vi "ESC UART.vi"() -> (0 "error out":errorcluster)   [LabVIEW 2022 SP3]
doc: "This example performs writes and reads on a serial port, as directed by the user. You can press the Write and Read buttons, and change the Read Count, while the example is running.\n\nThe parameters set for the serial port must match the parameters of the connected instrument or device. In this example, the Read Count parameter specifies the number of bytes that the serial port reads. If there were more bytes at the port than the specified number, those bytes would not be read. If there were less bytes at the port than the specified number, you would receive a timeout error.\n\nThis example expands upon the flow control options for XON and XOFF, allowing the user to choose those control characters. Also, the user can enable or disable a termination character. Some devices require a termination character in order to identify the end of command strings. Some devices send a termination character to signify the end of data to be read. This example shows how you can end the Read operation once a termination character is detected in the buffer and/or append a termination character at the end of the Write data."
uses:
  Program Files/National Instruments/LabVIEW 2022/examples/Instrument IO/Serial/support/Serial - Settings.ctl
  Sub_vis/Upload Data.ctl
  Globals/Meas_global.vi
  <vilib>/Instr/_visa.llb/VISA Configure Serial Port (Instr).vi
panel:
  out "Port Number":string
  out "Sampling Freq Hz":dbl
  out "Status Flag":dbl
  out "Offset":i32
  out "unsigned byte array":u8[](array[numeric])
  out "No Of Errors":i32
  out "N Count":i32
  out "Happy":bool
  out "Status":bool
  out "Motor Duty Cycle":dbl
  out "Throttle Duty Cycle":dbl
  out "RPM":dbl
  out "Bus Current":dbl
  out "Voltage":dbl
  out "ESC Temperature":dbl
  in  "Read Count/ No. of Bytes":u32=22
  in  "Serial Settings":T1={"baud rate"=115200, "data bits"=8, "parity"=enum."None", "stop bits"=10, "flow control"=0} {"flow control" items=["None"=0, "XON/XOFF"=1, "RTS/CTS"=2, "DTR/DSR"=4]; "stop bits" items=["1.0"=10, "1.5"=15, "2.0"=20]; "data bits" min=5 max=8 step=1; "baud rate" items=["75"=75, "110"=110, "134"=134, "150"=150, "300"=300, "600"=600, "1200"=1200, "1800"=1800, "2400"=2400, "4800"=4800, "7200"=7200, "9600"=9600, "14400"=14400, "19200"=19200, "28800"=28800, "38400"=38400, "56000"=56000, "57600"=57600, "115200"=115200, "128000"=128000, "230400"=230400]}
  # "Overview: Reads ESC Data from UART Pins + FTDI Cable (Converts UART to Serial). \nAPD HV PRO 240a:\nNumber of Bytes = 22\nBaudrate 115200\nData Bits = 8\nParity = None\nStop Bits = 1.0\nFlow Control = None"
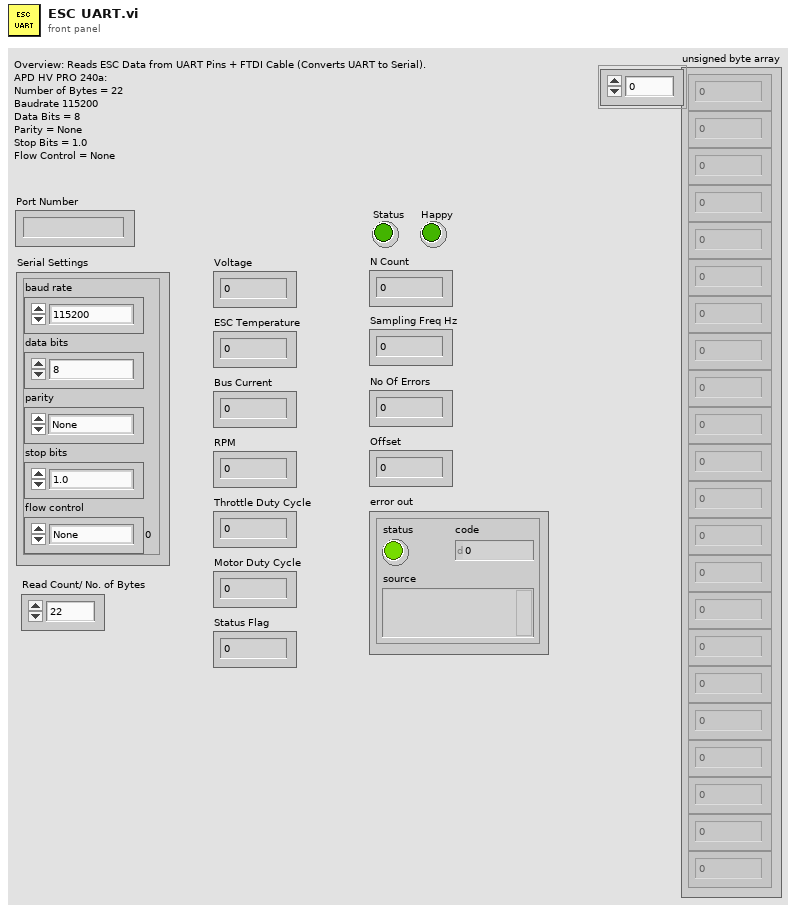
[diagram p1: front panel]
types:
  T1 = typedef "Serial - Settings.ctl" = cluster{"baud rate":u32, "data bits":u16, "parity":enum16{"None", "Odd", "Even", "Mark", "Space"}, "stop bits":u16, "flow control":u16}
  T2 = typedef "Setup.ctl" = enum16{"Run Program", "Show Setup", "Save Current Setup", "Setup Front Panel"}
  T3 = typedef "Upload Data.ctl" = enum16{"Voltage Array", "Time Trace Cluster"}
  T4 = typedef "Analysis_info_cluster.ctl" = cluster{"Colour":u32, "Inst type":T5, "Inst name":string, "Symbol":string, "Code name":string, "Extra Info":string, "Inst Array":T6, "Extra Titles":string[], "Extra Values":string[], "U":dbl, "u^2":dbl, "u^3":dbl, "u^4":dbl, "Skew_u":dbl, "Kurt_u":dbl, "Sd Error in Mean":dbl, "% u'/U":dbl, "X":dbl, "Y":dbl, "Z":dbl, "Timescale integral Estimate":dbl, "Sd Error in Variance":dbl, "Calib File":path, "Calib Constants":dbl[], "Output Position":bool, "Stats":enum16{"None", "Basic", "Full"}, "Av Sampling Rate":dbl, "Av No of Samples":dbl, "Total Meas Time (s)":dbl, "ADAM Ch Name":string, "Max value":dbl, "Min value":dbl, "Req Sample Rate Hz":dbl, "Sync Delay Time (s)":dbl, "Ch No":i16, "Device":string, "Use Latest Calib":bool, "Port":string, "Metadata Ch Names":string[], "Metadata Ch Values":string[], "Label":string}
  T5 = typedef "Inst_type.ctl" = enum16{"Raw voltage", "Raw with zero offsetting", "Propeller anemometer", "Pressure Transducer", "Pitot-static tube", "Hot wire", "Cross wire 1", "Cross wire 2", "Generic Linear", "Generic Polynomial", "Generic BackPoly", "Fast FID", "Thermocouple", "Cold wire", "Pulsed Wire", "LDA Vel", "LDA Tran time", "LDA Arr time", "Microphone"}
  T6 = typedef "Instrument_Array.ctl" = enum16{"PWA", "LDA", "Analogue"}
  T7 = typedef "Rendezvous RefNum" = refnum<k1>
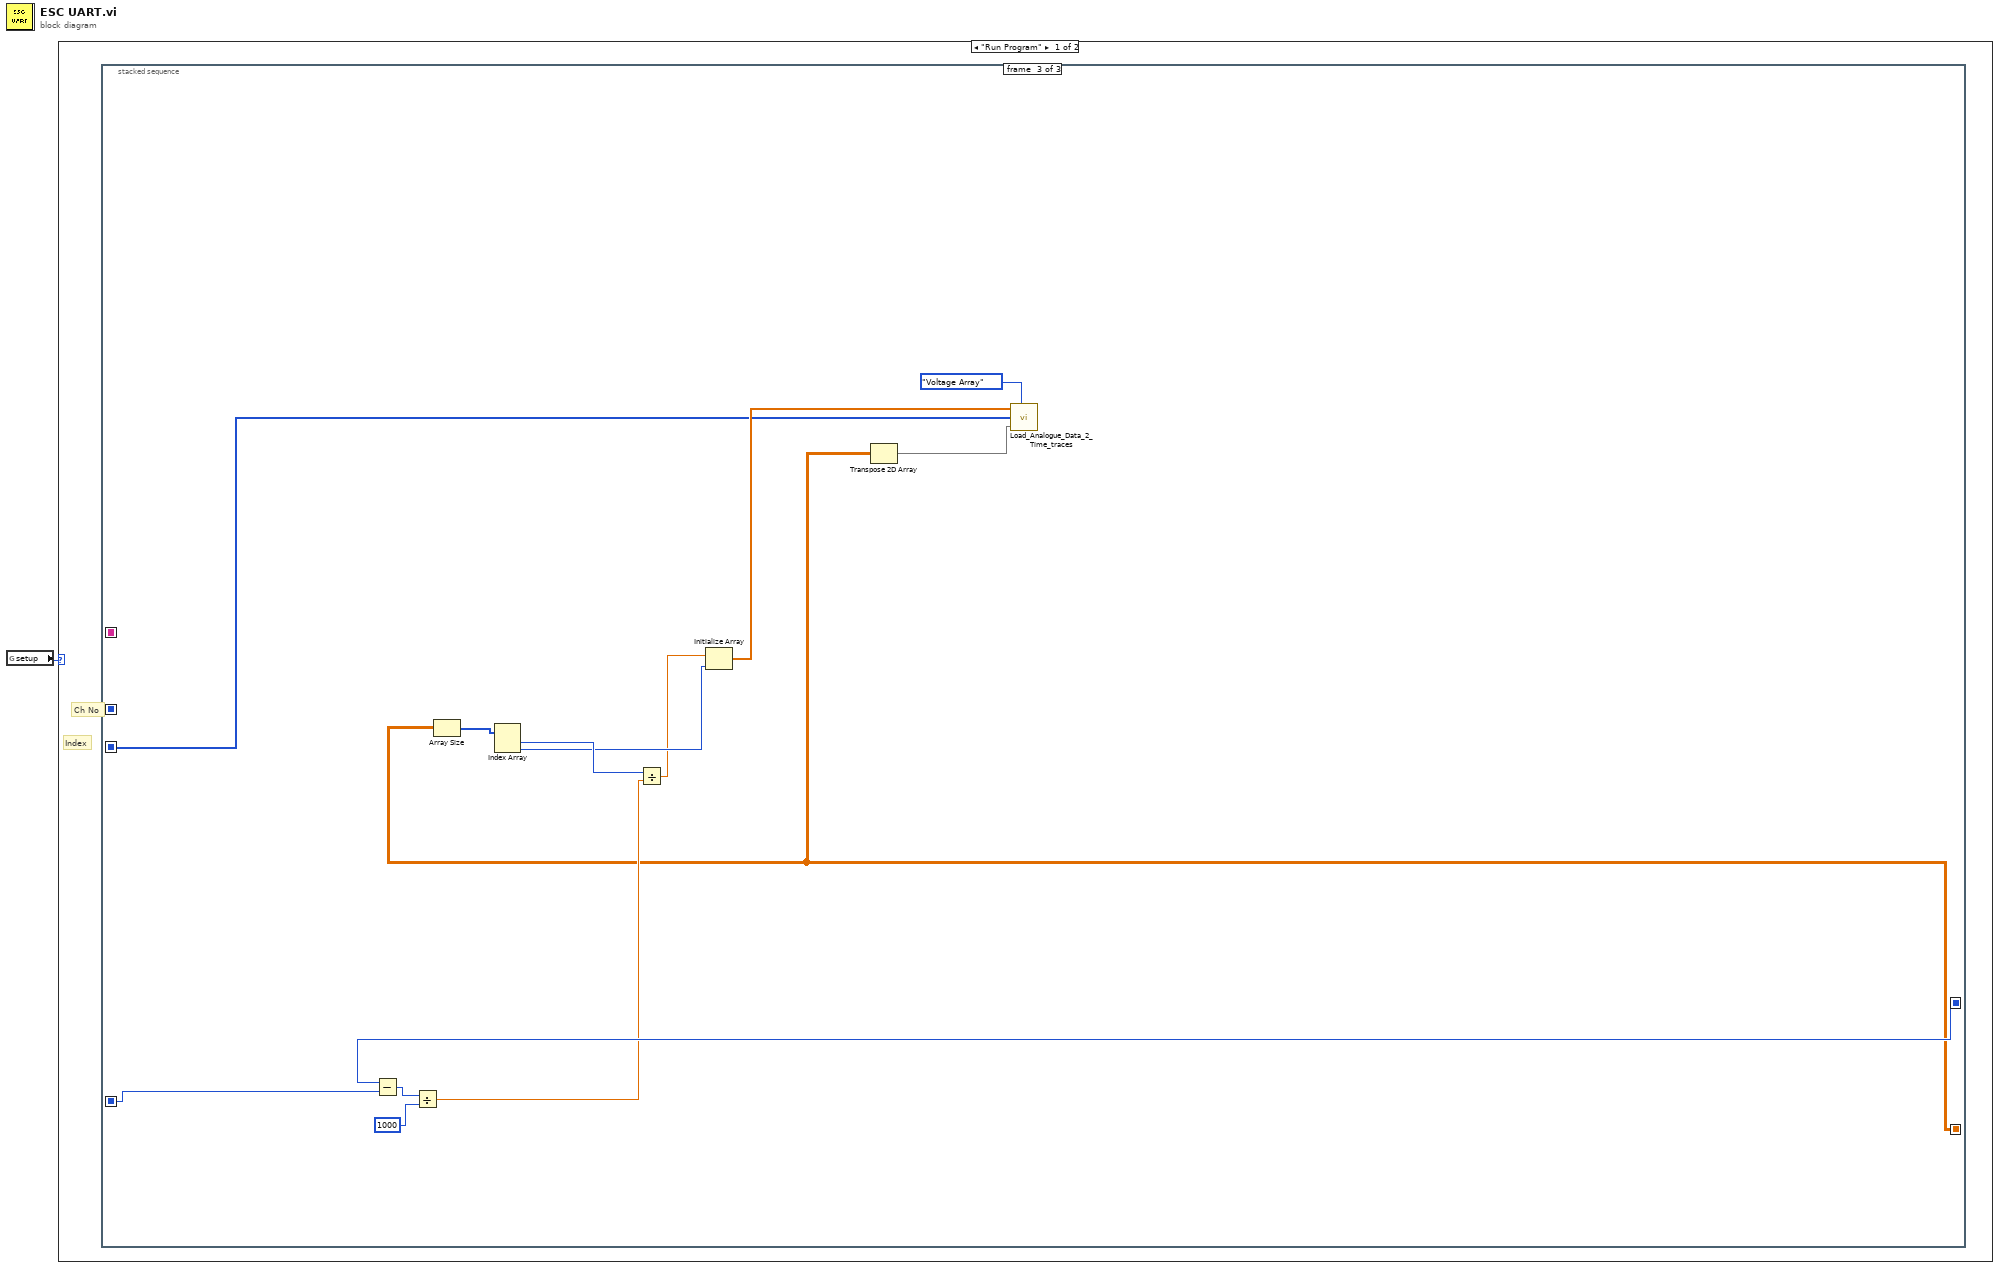
[diagram p0: block diagram]
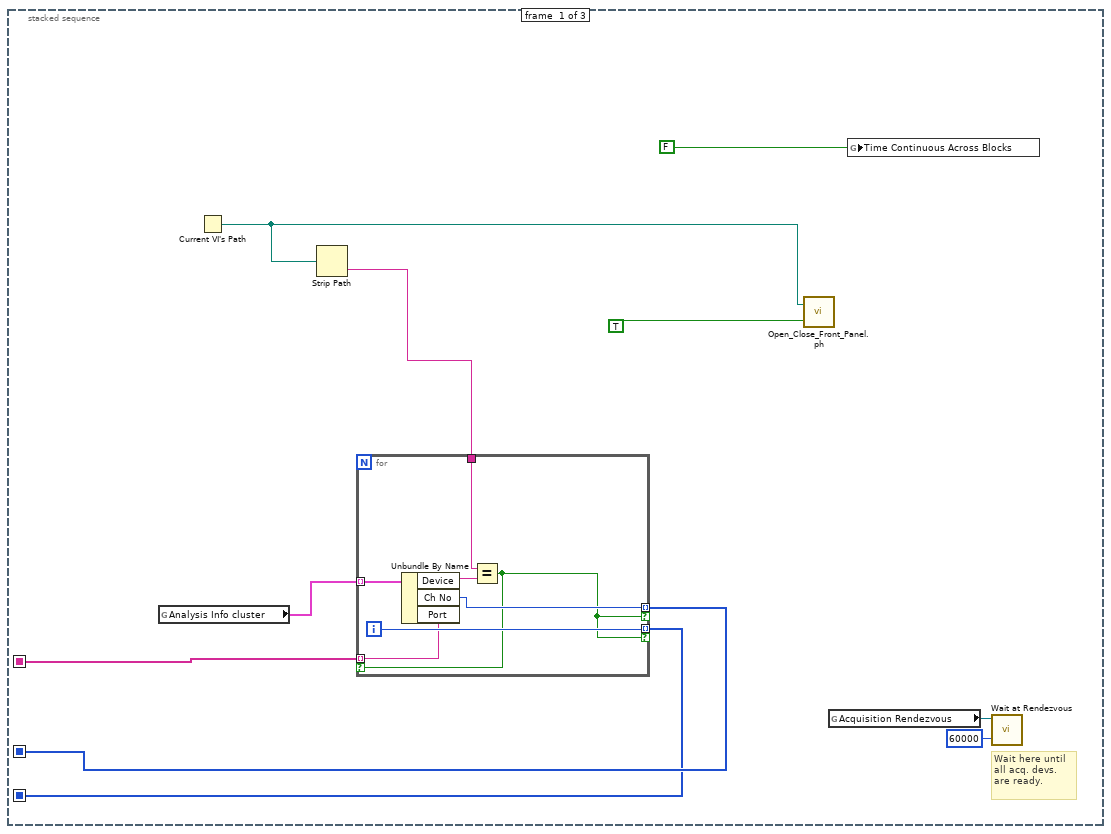
[diagram p2: hidden frame]
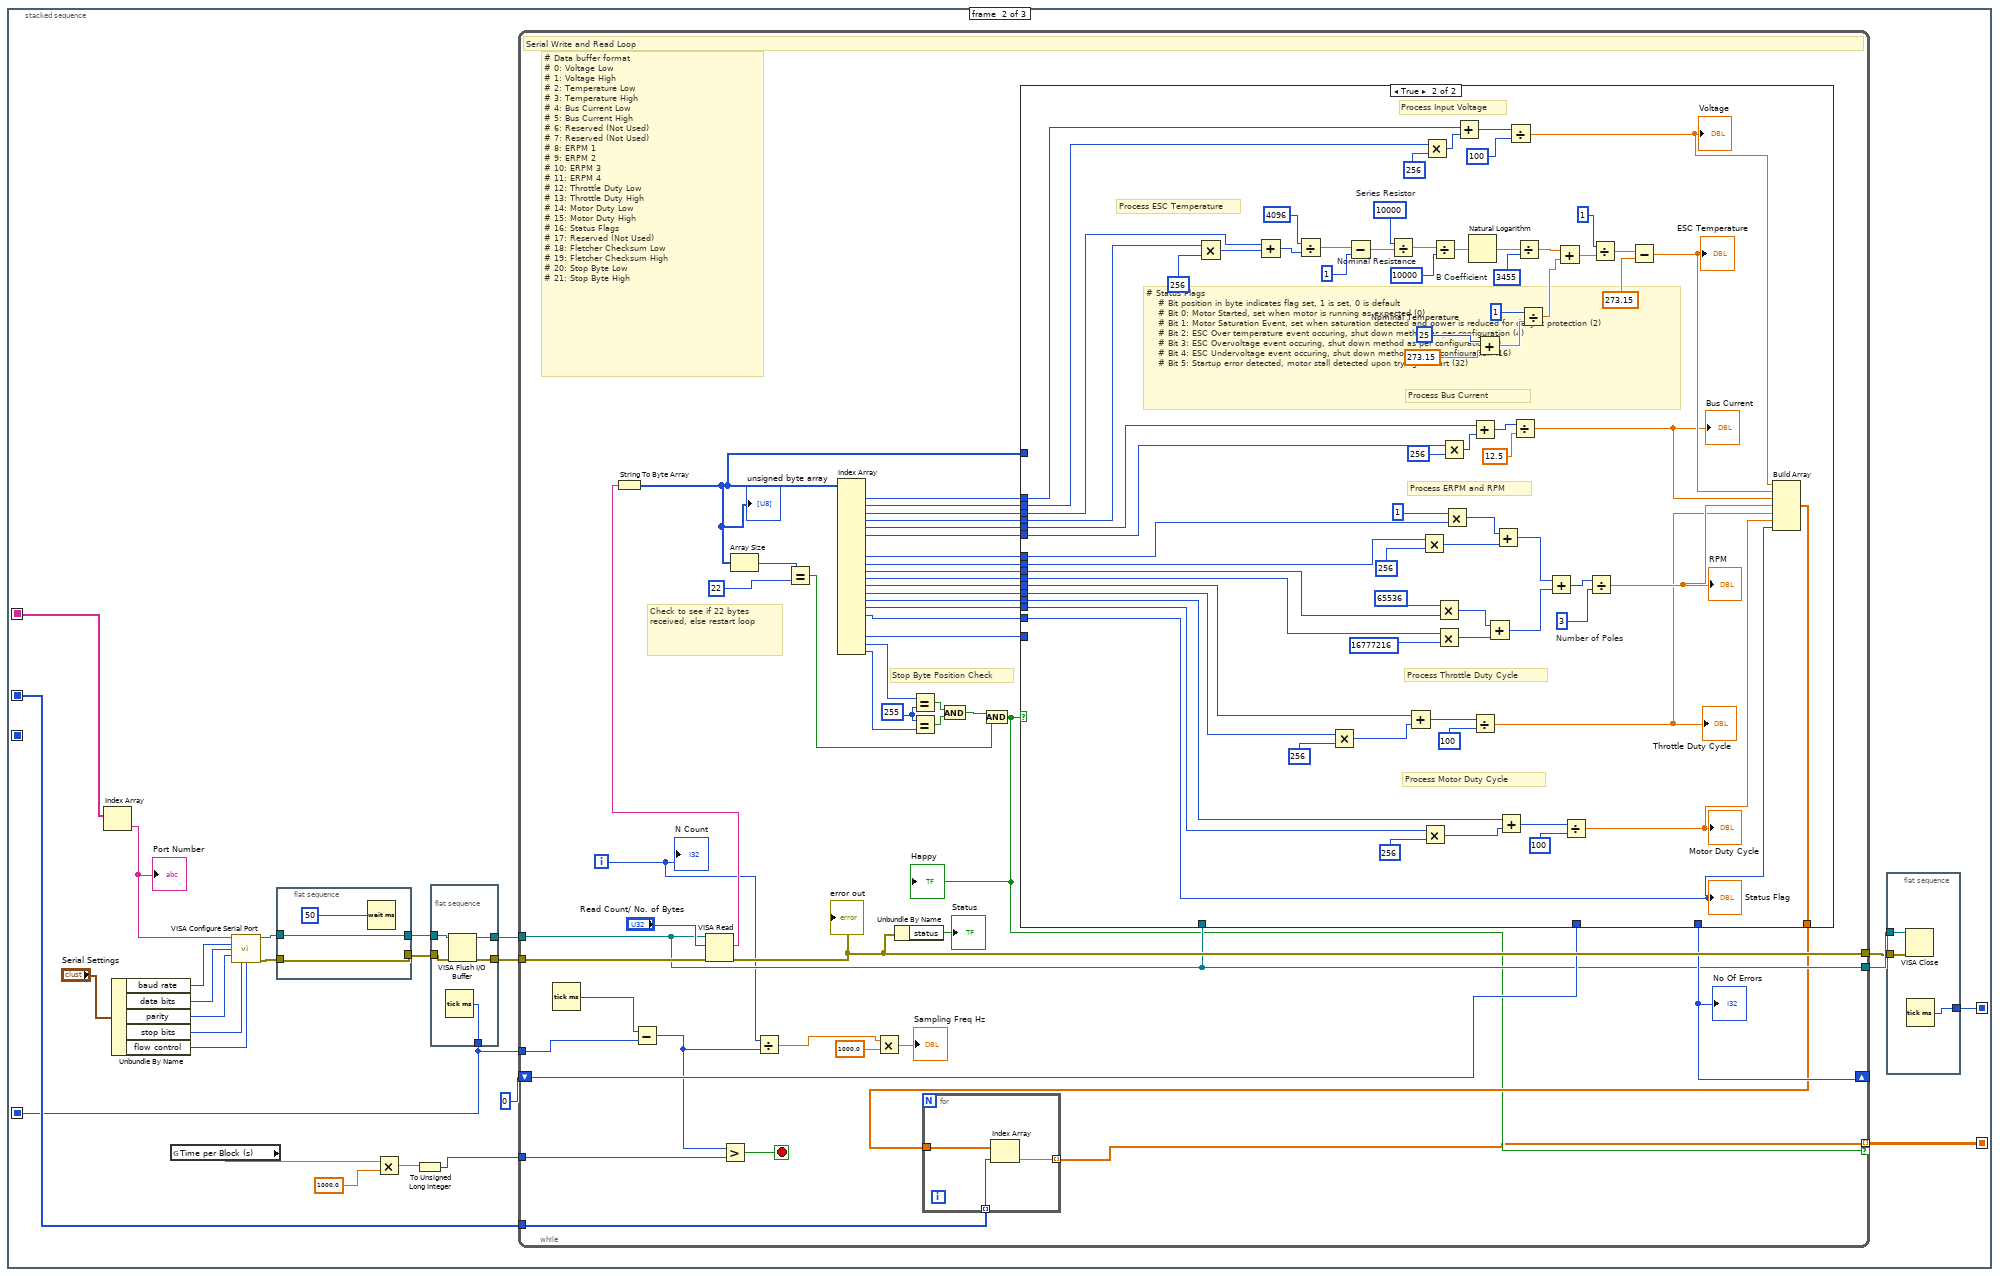
[diagram p3: hidden frame]
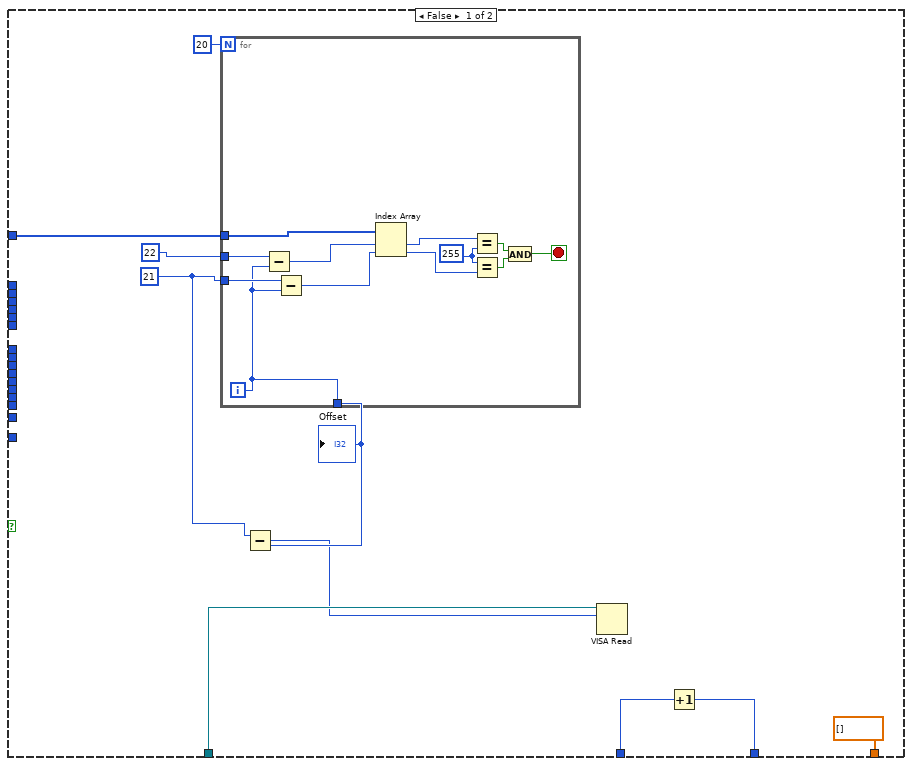
[diagram p4: hidden frame]
diagram:
  n1 = global read "Meas_global.vi" "setup"() -> (w1:T2)
  n2 = case shown="\"Run Program\"" w1 {
    frame "Run Program" {
      # "Index"
      # "Ch No"
      n3 = stacked-sequence {
        seq-local: [w4 _ _] -> [_ w27 _]
        seq-local: [_ w28 _] -> [_ _ w202]
        seq-local: [_ w22 _] -> [_ _ w213]
        seq-local: [_ w26 _] -> [_ _ w214]
        seq-local: [w3 _ _] -> [_ _ w204]
        seq-local: [w2 _ _] -> [_ w20 _]
        frame #0 {
          # "Wait here until all acq. devs. are ready."
          n4 = global read "Meas_global.vi" "Analysis Info cluster"() -> (w6:T4[])
          n5 = Current VI's Path() -> (path=w7:path)
          n6 = Strip Path(path=w7) -> (name=w5:string)  [unwired: 1 out]
          n7 = for {
            tunnel: w6 -> [w18] mode=indexing
            tunnel: w5 -> [w16]
            tunnel: [w15] -> w4 mode=indexing if=w12
            tunnel: [w14] -> w3 mode=indexing if=w12
            tunnel: [w13] -> w2 mode=indexing if=w12
            i -> [w14]
            n8 = Unbundle By Name(w18) -> ("Device"=w17:string, "Ch No"=w15:i16, "Port"=w13:string)
            n9 = Equal?(x=w16, y=w17) -> (x = y?=w12:bool)
          }
          n10 = call "Open_Close_Front_Panel.ph.vi"("openWindow (T)"=TRUE ("Front Panel Window:Open"), "VI path"=w7) -> ()  [unwired: 1 in, 1 out]
          n11 = global read "Meas_global.vi" "Acquisition Rendezvous"() -> (w8:T7)
          n12 = global write "Meas_global.vi" "Time Continuous Across Blocks"(FALSE ("Time Continuous across Blocks")) -> ()
          n13 = call <vilib>:"Wait at Rendezvous.vi"("ms timeout (-1)"=60000, "rendezvous"=w8) -> ()  [unwired: 3 in, 3 out]
        }
        frame #1 {
          n14 = Index Array(array=w20) -> (element=w19:string)  [unwired: 1 in]
          "Port Number" <- w19
          n15 = Unbundle By Name("Serial Settings") -> ("baud rate"=w40:u32, "data bits"=w41:u16, "parity"=w42:enum16{"None", "Odd", "Even", "Mark", "Space"}, "stop bits"=w43:u16, "flow control"=w38:u16)
          n16 = global read "Meas_global.vi" "Time per Block (s)"() -> (w25:dbl)
          n17 = call-poly "VISA Configure Serial Port"("VISA resource name"=w19, "baud rate (9600)"=w40, "data bits (8)"=w41, "parity (0:none)"=w42, "stop bits (10: 1 bit)"=w43, "flow control (0:none)"=w38) -> ("VISA resource name out"=w37:refnum<visa-resource-name>, "error out"=w36:errorcluster)  [unwired: 4 in, 4 out]
          n18 = flat-sequence {
            tunnel: w37 -> [w53]
            tunnel: [w53] -> w35
            tunnel: w36 -> [w52]
            tunnel: [w52] -> w32
            frame #0 {
              n19 = Wait (ms)(milliseconds to wait=50) -> ()  [unwired: 1 out]
            }
          }
          n20 = Multiply(x=w25, y=1000.0) -> (x*y=w23:dbl)
          n21 = To Unsigned Long Integer(number=w23) -> (unsigned 32bit integer=w21:u32)
          n22 = flat-sequence {
            tunnel: w35 -> [w51]
            tunnel: [w50] -> w34
            tunnel: [w49] -> w33
            tunnel: w32 -> [w48]
            tunnel: [w47] -> w22
            frame #0 {
              n23 = Tick Count (ms)() -> (millisecond timer value=w47:u32)
              n24 = VISA Flush I/O Buffer(VISA resource name=w51, error in (no error)=w48) -> (VISA resource name out=w50:refnum<visa-resource-name>, error out=w49:errorcluster)  [unwired: 1 in]
            }
          }
          n25 = while {
            tunnel: w33 -> [w93]
            tunnel: w34 -> [w68]
            tunnel: [w68] -> w31
            tunnel: [w74] -> w30
            shift-right: [w70] -> _
            shift-left: 0 -> [w71]
            tunnel: w27 -> [w65]
            tunnel: [w63] -> w28 mode=indexing if=w64
            tunnel: w22 -> [w62]
            tunnel: w21 -> [w61]
            i -> [w59]
            stop <- w60 stop-if-true
            w96 = u8 255 ("y")
            # "Stop Byte Position Check"
            # "Check to see if 22 bytes received, else restart loop"
            # "# Data buffer format\n# 0: Voltage Low \n# 1: Voltage High\n# 2: Temperature Low \n# 3: Temperature High\n# 4: Bus Current Low\n# 5: Bus Current High\n# 6: Reserved (Not Used)\n# 7: Reserved (Not Used)\n# 8: ERPM 1\n# 9: ERPM 2\n# 10: ERPM 3\n# 11: ERPM 4\n# 12: Throttle Duty Low\n# 13: Throttle Duty High\n# 14: Motor Duty Low\n# 15: Motor Duty High\n# 16: Status Flags\n# 17: Reserved (Not Used)\n# 18: Fletcher Checksum Low\n# 19: Fletcher Checksum High\n# 20: Stop Byte Low\n# 21: Stop Byte High"
            # "Serial Write and Read Loop"
            n26 = Tick Count (ms)() -> (millisecond timer value=w72:u32)
            n27 = Subtract(x=w72, y=w62) -> (x-y=w58:u32)
            n28 = VISA Read(VISA resource name=w68, byte count="Read Count/ No. of Bytes", error in (no error)=w93) -> (read buffer=w79:string, error out=w74:errorcluster)  [unwired: 2 out]
            "error out" <- w74
            n29 = String To Byte Array(string=w79) -> (unsigned byte array=w69:u8[])
            "unsigned byte array" <- w69
            n30 = Greater?(x=w58, y=w61) -> (0:w60:bool)
            n31 = Array Size(array=w69) -> (size(s)=w77:i32)
            n32 = Divide(x=w59, y=w58) -> (x/y=w56:dbl)
            n33 = Equal?(x=w77, y=22) -> (x = y?=w75:bool)
            n34 = Index Array(array=w69) -> (element #1=w90:u8, element #2=w91:u8, element #3=w100:u8, element #4=w101:u8, element #5=w88:u8, element #6=w89:u8, element #9=w84:u8, element #10=w87:u8, element #11=w86:u8, element #12=w85:u8, element #13=w83:u8, element #14=w82:u8, element #15=w81:u8, element #16=w80:u8, element #17=w67:u8, element #20=w92:u8, element #21=w95:u8, element #22=w97:u8)  [unwired: 22 in, 4 out]
            n35 = Multiply(x=w56, y=1000.0) -> (x*y=→"Sampling Freq Hz":dbl)
            n36 = Unbundle By Name(w74) -> ("status"=→"Status":bool)
            n37 = Equal?(x=w95, y=w96) -> (x = y?=w98:bool)
            n38 = Equal?(x=w96, y=w97) -> (x = y?=w99:bool)
            n39 = And(x=w98, y=w99) -> (x .and. y?=w76:bool)
            n40 = And(x=w76, y=w75) -> (x .and. y?=w64:bool)
            "Happy" <- w64
            n41 = case shown="True" w64 {
              tunnel: w101 -> [_ w200]
              tunnel: w100 -> [_ w199]
              tunnel: w92 -> [_ _]
              tunnel: w91 -> [_ w174]
              tunnel: w90 -> [_ w173]
              tunnel: w89 -> [_ w166]
              tunnel: w88 -> [_ w165]
              tunnel: w87 -> [_ w161]
              tunnel: w86 -> [_ w154]
              tunnel: w85 -> [_ w153]
              tunnel: w84 -> [_ w152]
              tunnel: w83 -> [_ w146]
              tunnel: w82 -> [_ w145]
              tunnel: w81 -> [_ w137]
              tunnel: w80 -> [_ w136]
              tunnel: w71 -> [w114 w135]
              tunnel: [w113 w135] -> w70
              tunnel: w69 -> [w112 _]
              tunnel: w68 -> [w109 _]
              tunnel: w67 -> [_ w128]
              tunnel: [dbl[] [] w127] -> w66
              frame False {
                w108 = 21 ("index")
                n42 = for {
                  N: 20 -> [_]
                  tunnel: w112 -> [w126]
                  tunnel: 22 ("index") -> [w125]
                  tunnel: w108 -> [w123]
                  tunnel: [w115] -> w107
                  i -> [w115]
                  stop <- w116 stop-if-true
                  w119 = u8 255 ("y")
                  n43 = Subtract(x=w125, y=w115) -> (x-y=w124:i32)
                  n44 = Subtract(x=w123, y=w115) -> (x-y=w122:i32)
                  n45 = Index Array(array=w126, index #1=w124, index #2=w122) -> (element #1=w118:u8, element #2=w117:u8)
                  n46 = Equal?(x=w118, y=w119) -> (x = y?=w120:bool)
                  n47 = Equal?(x=w119, y=w117) -> (x = y?=w121:bool)
                  n48 = And(x=w120, y=w121) -> (x .and. y?=w116:bool)
                }
                "Offset" <- w107
                n49 = Subtract(x=w108, y=w107) -> (x-y=w106:i32)
                n50 = VISA Read(VISA resource name=w109, byte count=w106) -> ()  [unwired: 1 in, 4 out]
                n51 = Increment(x=w114) -> (x+1=w113:i32)
              }
              frame True {
                w148 = 3  # Number of Poles
                w186 = 25  # Nominal Temperature
                w190 = 3455  # B Coefficient
                w191 = 10000  # Nominal Resistance
                w194 = 10000  # Series Resistor
                # "# Status Flags\n    # Bit position in byte indicates flag set, 1 is set, 0 is default\n    # Bit 0: Motor Started, set when motor is running as expected (0)\n    # Bit 1: Motor Saturation Event, set when saturation detected and power is reduced for desync protection (2)\n    # Bit 2: ESC Over temperature event occuring, shut down method as per configuration (4)\n    # Bit 3: ESC Overvoltage event occuring, shut down method as per configuration (8)\n    # Bit 4: ESC Undervoltage event occuring, shut down method as per configuration (16)\n    # Bit 5: Startup error detected, motor stall detected upon trying to start (32)"
                # "Process Motor Duty Cycle"
                # "Process Throttle Duty Cycle"
                # "Process ERPM and RPM"
                # "Process Bus Current"
                # "Process Input Voltage"
                # "Process ESC Temperature"
                n52 = Multiply(x=w200, y=256) -> (x*y=w176:i32)
                n53 = Add(x=w199, y=w176) -> (x+y=w198:i32)
                n54 = Divide(x=4096, y=w198) -> (x/y=w196:dbl)
                n55 = Multiply(x=w145, y=256) -> (x*y=w144:i32)
                n56 = Subtract(x=w196, y=1) -> (x-y=w193:dbl)
                n57 = Divide(x=w194, y=w193) -> (x/y=w192:dbl)
                n58 = Add(x=w146, y=w144) -> (x+y=w143:i32)
                n59 = Multiply(x=w161, y=256) -> (x*y=w159:i32)
                n60 = Multiply(x=w136, y=256) -> (x*y=w140:i32)
                n61 = Multiply(x=w174, y=256) -> (x*y=w172:i32)
                n62 = Divide(x=w192, y=w191) -> (x/y=w179:dbl)
                n63 = Multiply(x=65536 ("y"), y=w154) -> (x*y=w156:i32)
                n64 = Multiply(x=w153, y=16777216) -> (x*y=w155:i32)
                n65 = Multiply(x=w166, y=256) -> (x*y=w169:i32)
                n66 = Multiply(x=1 ("y"), y=w152) -> (x*y=w160:i32)
                n67 = Add(x=w173, y=w172) -> (x+y=w171:i32)
                n68 = Natural Logarithm(1:w179) -> (0:w178:dbl)
                n69 = Add(x=w165, y=w169) -> (x+y=w168:i32)
                n70 = Divide(x=w143, y=100) -> (x/y=w130:dbl)
                "Throttle Duty Cycle" <- w130
                n71 = Add(x=w186, y=273.15) -> (x+y=w185:dbl)
                n72 = Add(x=w156, y=w155) -> (x+y=w151:i32)
                n73 = Add(x=w160, y=w159) -> (x+y=w150:i32)
                n74 = Add(x=w137, y=w140) -> (x+y=w139:i32)
                n75 = Divide(x=w171, y=100) -> (x/y=w134:dbl)
                "Voltage" <- w134
                n76 = Divide(x=w168, y=12.5) -> (x/y=w132:dbl)
                "Bus Current" <- w132
                n77 = Divide(x=w178, y=w190) -> (x/y=w189:dbl)
                n78 = Divide(x=1, y=w185) -> (x/y=w184:dbl)
                n79 = Add(x=w150, y=w151) -> (x+y=w149:i32)
                n80 = Add(x=w189, y=w184) -> (x+y=w183:dbl)
                n81 = Divide(x=w139, y=100) -> (x/y=w129:dbl)
                "Motor Duty Cycle" <- w129
                n82 = Divide(x=w149, y=w148) -> (x/y=w131:dbl)
                "RPM" <- w131
                n83 = Divide(x=1, y=w183) -> (x/y=w181:dbl)
                n84 = Subtract(x=w181, y=273.15) -> (x-y=w133:dbl)
                "ESC Temperature" <- w133
                n85 = Build Array(w134, w133, w132, w131, w130, w129, w128) -> (w127:dbl[])
                "Status Flag" <- w128
              }
            }
            "No Of Errors" <- w70
            n86 = for {
              tunnel: w66 -> [w104]
              tunnel: w65 -> [w103] mode=indexing
              tunnel: [w102] -> w63 mode=indexing
              n87 = Index Array(array=w104, index=w103) -> (element=w102:dbl)
            }
            "N Count" <- w59
          }
          n88 = flat-sequence {
            tunnel: w31 -> [w46]
            tunnel: w30 -> [w45]
            tunnel: [w44] -> w26
            frame #0 {
              n89 = VISA Close(VISA resource name=w46, error in (no error)=w45) -> ()  [unwired: 1 out]
              n90 = Tick Count (ms)() -> (millisecond timer value=w44:u32)
            }
          }
        }
        frame #2 {
          n91 = Subtract(x=w214, y=w213) -> (x-y=w210:u32)
          n92 = Divide(x=w210, y=u32 1000) -> (x/y=w208:dbl)
          n93 = Array Size(array=w202) -> (size(s)=w212:i32[])
          n94 = Index Array(array=w212) -> (element #1=w211:i32, element #2=w207:i32)  [unwired: 2 in]
          n95 = Divide(x=w211, y=w208) -> (x/y=w206:dbl)
          n96 = Initialize Array(w206, w207) -> (w205:dbl[])
          n97 = Transpose 2D Array(2D array=w202) -> (transposed array=w201:dbl[][])
          n98 = call "Load_Analogue_Data_2_Time_traces.vi"("Sampling Rate (Hz)"=w205, "Mode"=Upload_Data."Voltage Array", "Index"=w204, "Voltage Array"=w201) -> ()  [unwired: 3 in]
        }
      }
    }
    frame "Show Setup", Default {
    }
  }
